vi "HEWH Get Agilent Data.vi"(7 "RLT Station Channels":T1, 8 "error in (no error)":errorcluster, 11 "Test Fixture Hardware":T3={"Power "={"Yokogawa"={"WT210"={"Sample Rate (1: 0.25s)"=1, "A Range (12: 20A)"=12, "V Range (6: 600V)"=4, "Power VISA Yokogawa WT210"="WT210"}, "WT500"={"Power VISA Yokogawa WT500"="WT500", "V Range (8: 1000V)"=0, "I Range (7: 40A)"=0, "Update Rate (3: 500ms)"=2}, "WT310_2"={"Sample Rate (1: 0.25s)"=1, "A Range (12: 20A)"=11, "V Range (6: 600V)"=4, "Power VISA Yokogawa WT310_2"="WT310_2"}, "WT310_3"={"Sample Rate (1: 0.25s)"=1, "A Range (12: 20A)"=11, "V Range (6: 600V)"=4, "Power VISA Yokogawa WT310_3"="WT310_3"}}, "Aplus"={"Aplus IP Address"="192.168.1.101", "Remote Port"=502, "Instrument"="APLUS", "Instr Driver Revision"="1.03.0053"}, "Power Limits"={"Crest Factor"={"Upper Limit"=1.49, "Lower Limit"=1.34}, "Harmonic Content"={"Uthd"=2.0}, "Voltage"={"% Error"=2.0}, "Stability"={"<1 Watt "={"Wattage"=1.0, "Slope (mW/H)"=10.0}, ">1 Watt"={"1%Power/Hour"=1.0}}}, "Nominal Voltage"=120, "Time Limit (s)"=10800.0, "Power Variation Limit (%)"=50.0, "Power Supply"={"Chroma 61605"="CHROMA", "Use Chroma?"=FALSE}}, "Weight Scale"={"Com Options"={"IND560Scale VISA"="LaurelMeter_Hot", "IP Address"="192.168.1.50", "Remote Port"=502, "Setra Scale VISA"="COM3", "GSE 350"="GSE350"}, "Select Scale"=""}, "Flow Rates"={"Laurel Cold IP Address"="", "Laurel Hot IP Address"="", "Hot Water Laurel VISA"="34972A_3", "Cold Water Laurel VISA"="MW100", "Remote Port"=0, "Laurel Communication Type"="", "Meters To Collect (Hot Cold)"="", "HOT Laurel Reference"=refnum, "COLD Laurel Reference"=refnum}, "Analog Data"={"Agilent"={"Agilent 34972_1"="34972A_1", "Agilent 34972_2"="34972A_2", "Agilent 34972_3"="34972A_3", "Agilent 34972_4"="34972A_3", "Agilent 34972_5"="34972A_3", "Agilent 34972_6"="34972A_3", "Agilent Gain"=0.0, "TC Type (K,J,T)"="", "Instrument IDN?"="", "TC Channels-List"="", "Analog Channels-List"="", "Agilent Cluster Array"=[], "TC Channels-List 2"="", "Analog Channels-List 2"=""}, "Yokogawa"={"MW100"="MW100", "Intellifaucet"=FALSE}, "Select Analog"="", "TC Coefficients"={"TC Coefficients 1"=[], "TC Coefficients 2"=[], "TC Coefficients 3"=[], "TC Coefficients 4"=[], "TC Coefficients 5"=[], "TC Coefficients 6"=[], "TC Coefficients 7"=[]}, "NI Tasks (Dryer DOE)"=["TC Temps-Module 1", "TC Temps-Module 2", "TC Temps-Module 3", "TC Temps-Module 4", "TC Temps-Module 5", "Gas and Temp-Module 6", "AC_DC Events-Module 7"], "Laurel Analog"={"Laurel IP (Water Temp)"="", "Laurel IP (Pressure)"=""}}, "ITHX-Temp Humidity"={"IP Address 1"="", "Remote Port"=0, "IP Address 2"="", "IP Address 3"=""}, "Gas Meter COM Ports"={"Gas Meter 1"="COM3", "Gas Meter 2"="COM4", "Gas Meter 3"="COM5", "Gas Meter 4"="COM6", "Gas Meter 5"="COM7", "Gas Meter 6"="COM8"}, "Barometric Pressure"={"HEISE 901A"="HEISE", "Use Barometer?"=FALSE}} {"Power"."Yokogawa"."WT310_3"."V Range (6: 600V)" items=["Auto", "15V", "30V", "60V", "150V", "300V", "600V"]; "Power"."Yokogawa"."WT310_3"."A Range (12: 20A)" items=["Auto", "5mA", "10mA", "20mA", "50mA", "100mA", "200mA", "0.5A", "1A", "2A", "5A", "10A", "20A", "50mV", "100mV", "200mV", "2.5V", "5V", "10V"]; "Power"."Yokogawa"."WT310_3"."Sample Rate (1: 0.25s)" items=["0.1s", "0.25s", "0.5s", "1s", "2s", "5s"]; "Power"."Yokogawa"."WT310_2"."V Range (6: 600V)" items=["Auto", "15V", "30V", "60V", "150V", "300V", "600V"]; "Power"."Yokogawa"."WT310_2"."A Range (12: 20A)" items=["Auto", "5mA", "10mA", "20mA", "50mA", "100mA", "200mA", "0.5A", "1A", "2A", "5A", "10A", "20A", "50mV", "100mV", "200mV", "2.5V", "5V", "10V"]; "Power"."Yokogawa"."WT310_2"."Sample Rate (1: 0.25s)" items=["0.1s", "0.25s", "0.5s", "1s", "2s", "5s"]; "Power"."Yokogawa"."WT500"."Update Rate (3: 500ms)" items=["-", "100ms", "200ms", "500ms", "1s", "2s", "5s"]; "Power"."Yokogawa"."WT500"."I Range (7: 40A)" items=["AUTO", "500 mA", "1 A", "2 A", "5 A", "10 A", "20 A", "40 A", "S-AUTO", "50 mV", "100 mV", "200 mV", "500 mV", "1 V", "2 V", "5 V", "10 V", "250 mA", "500 mA", "1 A", "2.5 A", "5 A", "10 A", "20 A", "25 mV", "50 mV", "100 mV", "250 mV", "500 mV", "1 V", "2.5 V", "5 V"]; "Power"."Yokogawa"."WT500"."V Range (8: 1000V)" items=["AUTO", "15", "30", "60", "100", "150", "300", "600", "1000", "7.5", "15", "30", "50", "75", "150", "300", "500"]; "Power"."Yokogawa"."WT210"."V Range (6: 600V)" items=["Auto", "15V", "30V", "60V", "150V", "300V", "600V"]; "Power"."Yokogawa"."WT210"."A Range (12: 20A)" items=["Auto", "5mA", "10mA", "20mA", "50mA", "100mA", "200mA", "0.5A", "1A", "2A", "5A", "10A", "20A", "50mV", "100mV", "200mV", "2.5V", "5V", "10V"]; "Power"."Yokogawa"."WT210"."Sample Rate (1: 0.25s)" items=["0.1s", "0.25s", "0.5s", "1s", "2s", "5s"]}) -> (0 "error out":errorcluster, 2 "Agilent Calibrated Cluster Array":T2[](array[typedef]), 3 "Agilent Data":string[][](array[string]))   [LabVIEW 2016]
uses:
  Washer DOE/Type Definitions/DOE Test Fixture Hardware.ctl
  Utility/Type Definitions/UTILITY Power Inputs Control.ctl
  Drivers/IND560 Scale Monitor/Type Definitions/IND560 Configuration.ctl
  Type Definitions/HEWH Agilent Cluster.ctl
  Utility/Type Definitions/UTILITY TC Coefficients.ctl
  Drivers/Omega FMA-1600A Series Gas Flow Meter/Type Definitions/FMA1600A COM Ports.ctl
  Type Definitions/HEWH RLT MW100 Station Channels.ctl
panel:
  out "Analog Data.Agilent.Agilent Cluster Array":T2[](array[typedef])
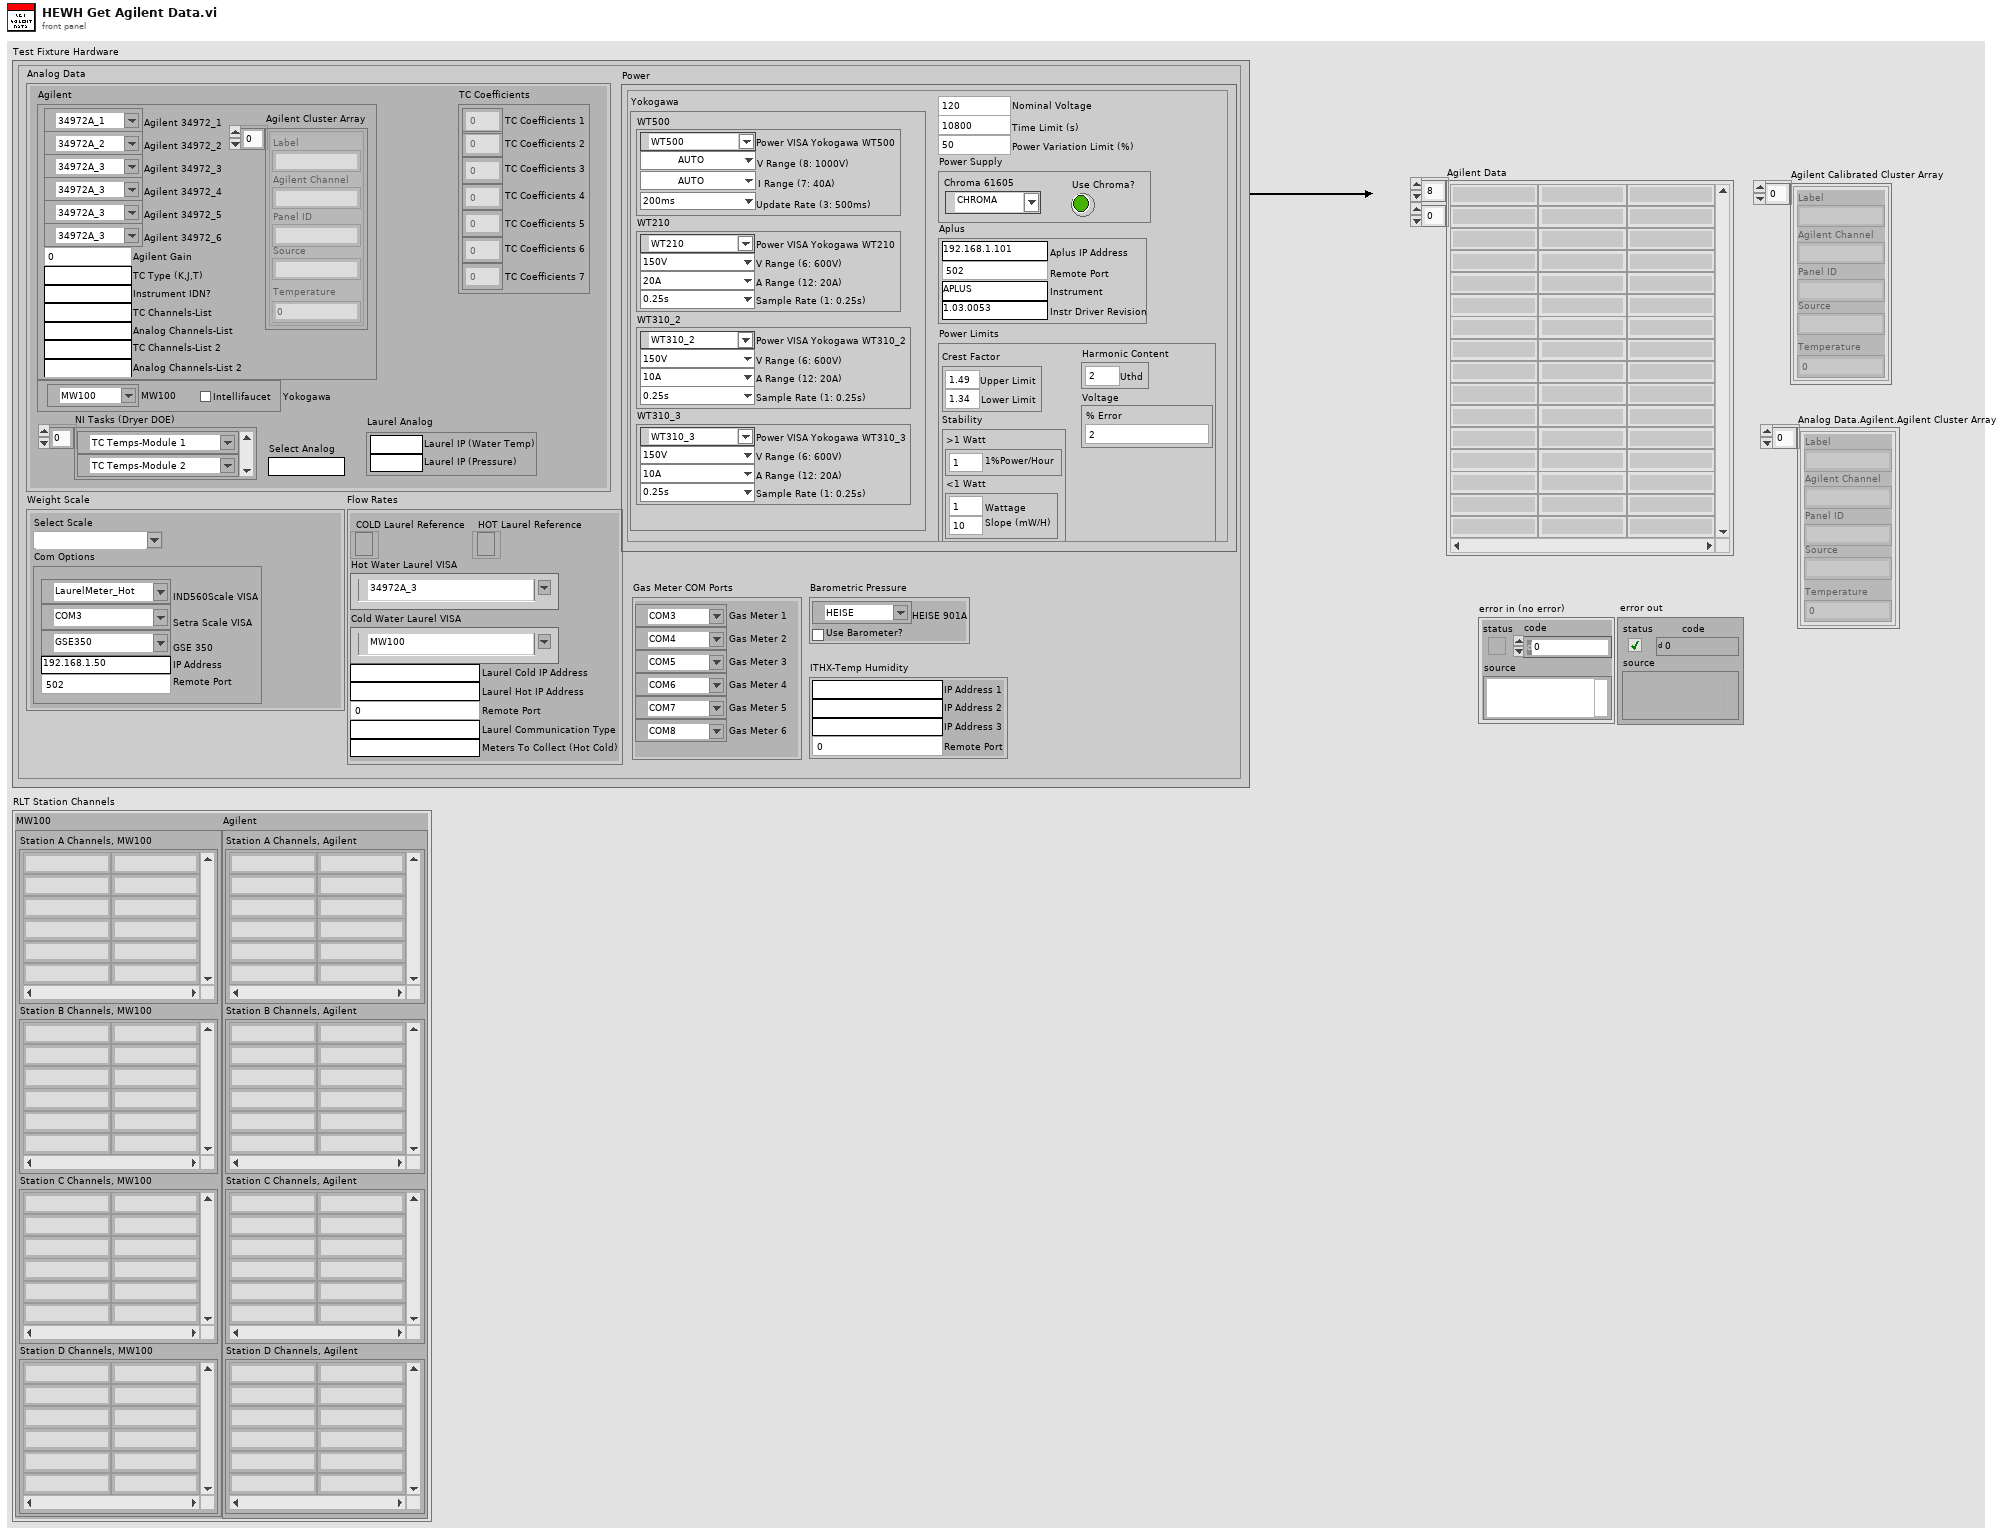
[diagram p1: front panel]
types:
  T1 = typedef "HEWH RLT MW100 Station Channels.ctl" = cluster{"MW100":cluster{"Station A Channels, MW100":string[][], "Station B Channels, MW100":string[][], "Station C Channels, MW100":string[][], "Station D Channels, MW100":string[][]}, "Agilent":cluster{"Station A Channels, Agilent":string[][], "Station B Channels, Agilent":string[][], "Station C Channels, Agilent":string[][], "Station D Channels, Agilent":string[][]}}
  T2 = typedef "HEWH Agilent Cluster.ctl" = cluster{"Label":string, "Agilent Channel":string, "Panel ID":string, "Source":string, "Temperature":dbl}
  T3 = typedef "DOE Test Fixture Hardware.ctl" = cluster{"Power ":T4, "Weight Scale":cluster{"Com Options":T5, "Select Scale":string}, "Flow Rates":cluster{"Laurel Cold IP Address":string, "Laurel Hot IP Address":string, "Hot Water Laurel VISA":refnum<visa-resource-name>, "Cold Water Laurel VISA":refnum<visa-resource-name>, "Remote Port":u16, "Laurel Communication Type":string, "Meters To Collect (Hot Cold)":string, "HOT Laurel Reference":refnum<k5>, "COLD Laurel Reference":refnum<k5>}, "Analog Data":cluster{"Agilent":cluster{"Agilent 34972_1":refnum<visa-resource-name>, "Agilent 34972_2":refnum<visa-resource-name>, "Agilent 34972_3":refnum<visa-resource-name>, "Agilent 34972_4":refnum<visa-resource-name>, "Agilent 34972_5":refnum<visa-resource-name>, "Agilent 34972_6":refnum<visa-resource-name>, "Agilent Gain":dbl, "TC Type (K,J,T)":string, "Instrument IDN?":string, "TC Channels-List":string, "Analog Channels-List":string, "Agilent Cluster Array":T2[], "TC Channels-List 2":string, "Analog Channels-List 2":string}, "Yokogawa":cluster{"MW100":refnum<visa-resource-name>, "Intellifaucet":bool}, "Select Analog":string, "TC Coefficients":T6, "NI Tasks (Dryer DOE)":refnum<k21>[], "Laurel Analog":cluster{"Laurel IP (Water Temp)":string, "Laurel IP (Pressure)":string}}, "ITHX-Temp Humidity":cluster{"IP Address 1":string, "Remote Port":u16, "IP Address 2":string, "IP Address 3":string}, "Gas Meter COM Ports":T7, "Barometric Pressure":cluster{"HEISE 901A":refnum<visa-resource-name>, "Use Barometer?":bool}}
  T4 = typedef "UTILITY Power Inputs Control.ctl" = cluster{"Yokogawa":cluster{"WT210":cluster{"Sample Rate (1: 0.25s)":i32, "A Range (12: 20A)":i32, "V Range (6: 600V)":i32, "Power VISA Yokogawa WT210":refnum<visa-resource-name>}, "WT500":cluster{"Power VISA Yokogawa WT500":refnum<visa-resource-name>, "V Range (8: 1000V)":i32, "I Range (7: 40A)":i32, "Update Rate (3: 500ms)":i32}, "WT310_2":cluster{"Sample Rate (1: 0.25s)":i32, "A Range (12: 20A)":i32, "V Range (6: 600V)":i32, "Power VISA Yokogawa WT310_2":refnum<visa-resource-name>}, "WT310_3":cluster{"Sample Rate (1: 0.25s)":i32, "A Range (12: 20A)":i32, "V Range (6: 600V)":i32, "Power VISA Yokogawa WT310_3":refnum<visa-resource-name>}}, "Aplus":cluster{"Aplus IP Address":string, "Remote Port":i32, "Instrument":string, "Instr Driver Revision":string}, "Power Limits":cluster{"Crest Factor":cluster{"Upper Limit":dbl, "Lower Limit":dbl}, "Harmonic Content":cluster{"Uthd":dbl}, "Voltage":cluster{"% Error":dbl}, "Stability":cluster{"<1 Watt ":cluster{"Wattage":dbl, "Slope (mW/H)":dbl}, ">1 Watt":cluster{"1%Power/Hour":dbl}}}, "Nominal Voltage":i32, "Time Limit (s)":dbl, "Power Variation Limit (%)":dbl, "Power Supply":cluster{"Chroma 61605":refnum<visa-resource-name>, "Use Chroma?":bool}}
  T5 = typedef "IND560 Configuration.ctl" = cluster{"IND560Scale VISA":refnum<visa-resource-name>, "IP Address":string, "Remote Port":u16, "Setra Scale VISA":refnum<visa-resource-name>, "GSE 350":refnum<visa-resource-name>}
  T6 = typedef "UTILITY TC Coefficients.ctl" = cluster{"TC Coefficients 1":dbl[], "TC Coefficients 2":dbl[], "TC Coefficients 3":dbl[], "TC Coefficients 4":dbl[], "TC Coefficients 5":dbl[], "TC Coefficients 6":dbl[], "TC Coefficients 7":dbl[]}
  T7 = typedef "FMA1600A COM Ports.ctl" = cluster{"Gas Meter 1":refnum<visa-resource-name>, "Gas Meter 2":refnum<visa-resource-name>, "Gas Meter 3":refnum<visa-resource-name>, "Gas Meter 4":refnum<visa-resource-name>, "Gas Meter 5":refnum<visa-resource-name>, "Gas Meter 6":refnum<visa-resource-name>}
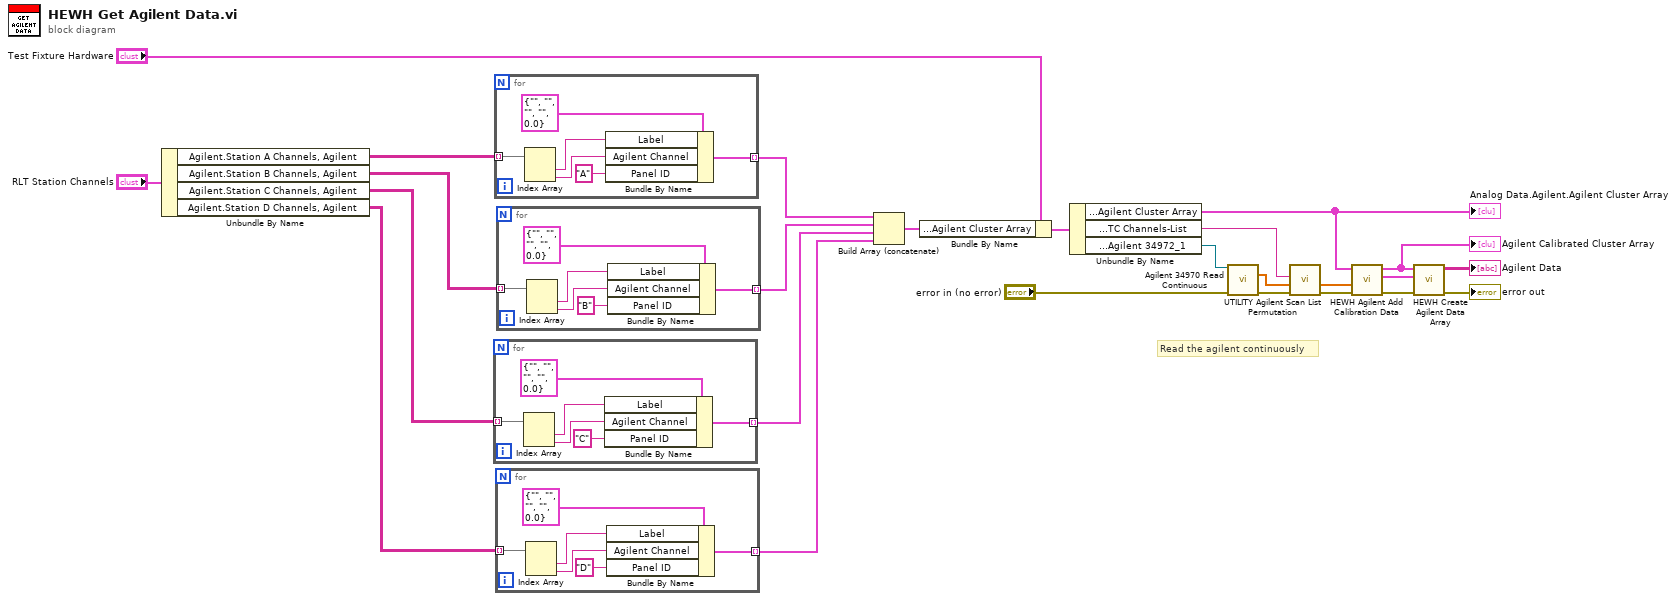
[diagram p0: block diagram]
diagram:
  # "Read the agilent continuously"
  n1 = Unbundle By Name("RLT Station Channels") -> ("Agilent.Station A Channels, Agilent"=w24:string[][], "Agilent.Station B Channels, Agilent"=w23:string[][], "Agilent.Station C Channels, Agilent"=w22:string[][], "Agilent.Station D Channels, Agilent"=w21:string[][])
  n2 = for {
    tunnel: w22 -> [w31] mode=indexing
    tunnel: [w26] -> w18 mode=indexing
    n3 = Index Array(array=w31) -> (element #1=w29:string, element #2=w28:string)  [unwired: 2 in]
    n4 = Bundle By Name(cluster=T2 {"Label"="", "Agilent Channel"="", "Panel ID"="", "Source"="", "Temperature"=0.0} ("Agilent Cluster"), "Label"=w29, "Agilent Channel"=w28, "Panel ID"="C") -> (w26:T2)
  }
  n5 = for {
    tunnel: w24 -> [w37] mode=indexing
    tunnel: [w32] -> w20 mode=indexing
    n6 = Index Array(array=w37) -> (element #1=w35:string, element #2=w34:string)  [unwired: 2 in]
    n7 = Bundle By Name(cluster=T2 {"Label"="", "Agilent Channel"="", "Panel ID"="", "Source"="", "Temperature"=0.0} ("Agilent Cluster"), "Label"=w35, "Agilent Channel"=w34, "Panel ID"="A") -> (w32:T2)
  }
  n8 = for {
    tunnel: w21 -> [w43] mode=indexing
    tunnel: [w38] -> w17 mode=indexing
    n9 = Index Array(array=w43) -> (element #1=w41:string, element #2=w40:string)  [unwired: 2 in]
    n10 = Bundle By Name(cluster=T2 {"Label"="", "Agilent Channel"="", "Panel ID"="", "Source"="", "Temperature"=0.0} ("Agilent Cluster"), "Label"=w41, "Agilent Channel"=w40, "Panel ID"="D") -> (w38:T2)
  }
  n11 = for {
    tunnel: w23 -> [w49] mode=indexing
    tunnel: [w44] -> w19 mode=indexing
    n12 = Index Array(array=w49) -> (element #1=w47:string, element #2=w46:string)  [unwired: 2 in]
    n13 = Bundle By Name(cluster=T2 {"Label"="", "Agilent Channel"="", "Panel ID"="", "Source"="", "Temperature"=0.0} ("Agilent Cluster"), "Label"=w47, "Agilent Channel"=w46, "Panel ID"="B") -> (w44:T2)
  }
  n14 = Build Array (concatenate)(w20, w19, w18, w17) -> (w1:T2[])
  n15 = Bundle By Name(cluster="Test Fixture Hardware", "Analog Data.Agilent.Agilent Cluster Array"=w1) -> (w2:T3)
  n16 = Unbundle By Name(w2) -> ("Analog Data.Agilent.Agilent Cluster Array"=w11:T2[], "Analog Data.Agilent.TC Channels-List"=w10:string, "Analog Data.Agilent.Agilent 34972_1"=w9:refnum<visa-resource-name>)
  "Analog Data.Agilent.Agilent Cluster Array" <- w11
  n17 = call "Agilent 34970 Read Continuous.vi"("VISA Resource Name"=w9, "error in (no error)"="error in (no error)") -> ("Output Array"=w12:dbl[], "error out"=w8:errorcluster)  [unwired: 10 in, 2 out]
  n18 = call "UTILITY Agilent Scan List Permutation.vi"("Error In"=w8, "Input Data Array"=w12, "Agilent Scan List"=w10) -> ("Error Out"=w7:errorcluster, "Output Data Permutation"=w4:dbl[])  [unwired: 6 in, 1 out]
  n19 = call "HEWH Agilent Add Calibration Data.vi"("Error In"=w7, "Sorted Agilent Data"=w4, "Agilent Cluster Array"=w11) -> ("Error Out"=w5:errorcluster, "Agilent Raw Cluster Array"=w15:T2[], "Agilent Calibrated Cluster Array"=w14:T2[])  [unwired: 6 in]
  "Agilent Calibrated Cluster Array" <- w14
  n20 = call "HEWH Create Agilent Data Array.vi"("Error In"=w5, "Agilent Raw Cluster Array"=w15, "Agilent Calibrated Cluster Array"=w14) -> ("Error Out"=→"error out":errorcluster, "Agilent Data(Label,Channel,Data)"=→"Agilent Data":string[][])  [unwired: 7 in]
